vi "stringToDatetime.vi"(9 "input string":string) -> (1 "date/time string":string, 3 "sqltime string":string, 4 "Shift":string, 6 "ShiftDate":string)   [LabVIEW 2012]
uses:
  <vilib>/Utility/miscctls.llb/LVDateTimeRec.ctl
panel:
  in  "date time rec":T1
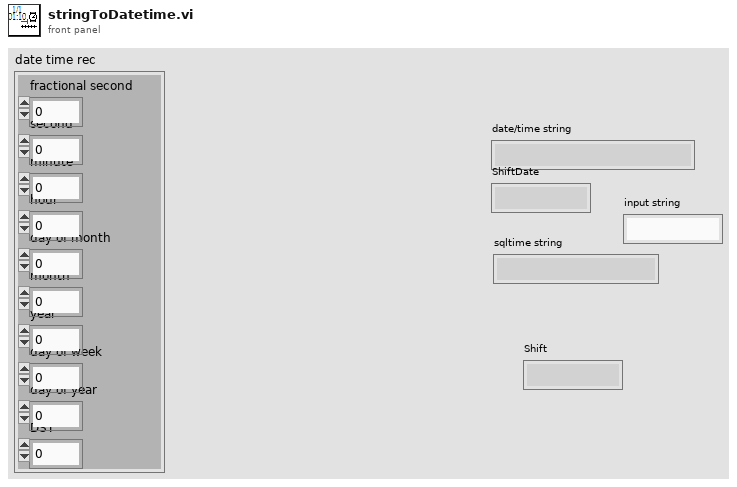
[diagram p1: front panel]
types:
  T1 = typedef "LVDateTimeRec.ctl" = cluster{"fractional second":dbl, "second":i32, "minute":i32, "hour":i32, "day of month":i32, "month":i32, "year":i32, "day of week":i32, "day of year":i32, "DST":i32}
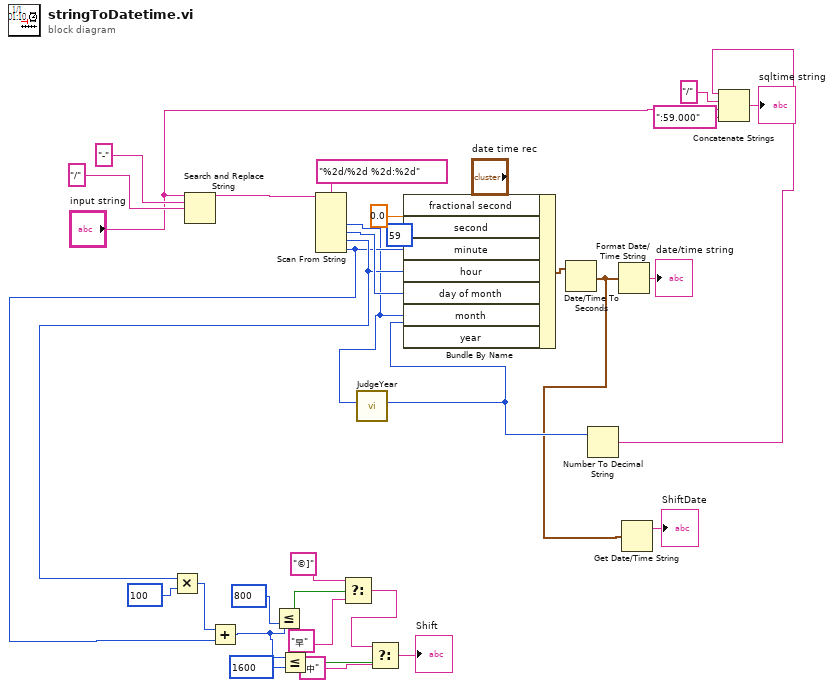
[diagram p0: block diagram]
diagram:
  n1 = Search and Replace String(input string="input string", search string="-", replace string="/" ("replace string (\"\")")) -> (result string=w24:string)  [unwired: 5 in, 3 out]
  n2 = Scan From String(format string="%2d/%2d %2d:%2d", input string=w24) -> (output 1=w3:i32, output 2=w28:i32, output 3=w8:i32, output 4=w7:i32)  [unwired: 6 in, 3 out]
  n3 = Multiply(x=w8, y=100) -> (x*y=w17:i32)
  n4 = Add(x=w17, y=w7) -> (x+y=w10:i32)
  n5 = Less Or Equal?(x=w10, y=800) -> (x <= y?=w4:bool)
  n6 = Less Or Equal?(x=w10, y=1600) -> (x <= y?=w12:bool)
  n7 = Select(t="©]", s=w4, f="早") -> (s? t:f=w9:string)
  n8 = call "JudgeYear.vi"("DataMonth"=w3) -> ("DataYear"=w2:i32)  [unwired: 10 in]
  n9 = Select(t=w9, s=w12, f="中") -> (s? t:f=→"Shift":string)
  n10 = Bundle By Name(cluster="date time rec", "fractional second"=0.0, "second"=59, "minute"=w7, "hour"=w8, "day of month"=w28, "month"=w3, "year"=w2) -> (w30:T1)
  n11 = Date/Time To Seconds(2:w30) -> (0:w1:timestamp)  [unwired: 1 in]
  n12 = Number To Decimal String(number=w2) -> (decimal integer string=w23:string)  [unwired: 1 in]
  n13 = Format Date/Time String(seconds (now)=w1) -> (date/time string=→"date/time string":string)  [unwired: 2 in]
  n14 = Get Date/Time String(seconds (now)=w1) -> (date string=→"ShiftDate":string)  [unwired: 2 in, 1 out]
  n15 = Concatenate Strings(w23, "/" ("string"), "input string", ":59.000" ("string")) -> (→"sqltime string":string)
